vi "Open Handle.vi"(8 "error in (no error)":errorcluster) -> (0 "error out":errorcluster, 3 "Refnum out":T1)   [LabVIEW 2018]
uses:
  <vilib>/httpClient/ClientHandle.ctl
  <vilib>/httpClient/LabVIEWHTTPClient.lvlib
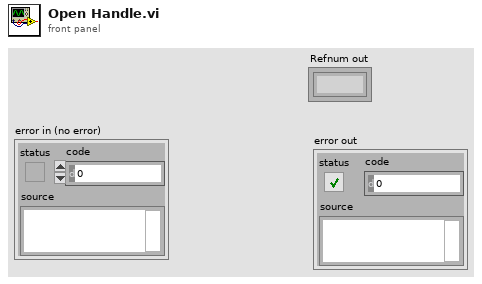
[diagram p1: front panel]
types:
  T1 = typedef "LabVIEWHTTPClient.lvlib/ClientHandle.ctl" = refnum<k1>
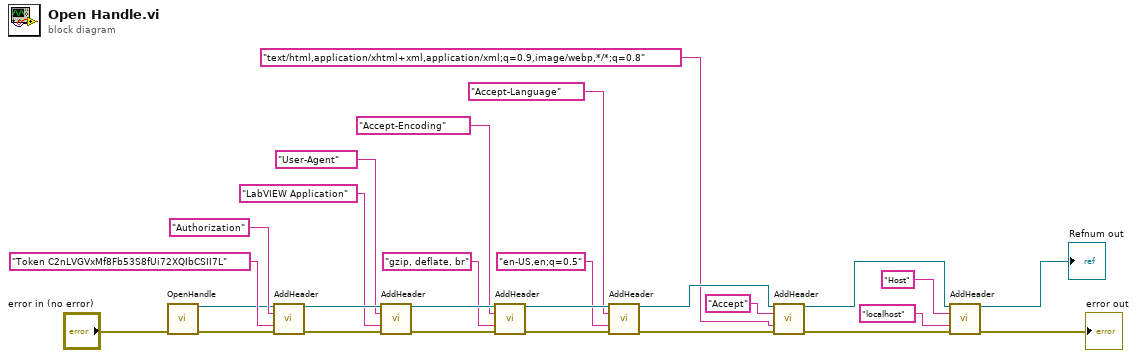
[diagram p0: block diagram]
diagram:
  n1 = call <vilib>:"OpenHandle.vi"("error in (no error)"="error in (no error)") -> ("client handle out"=w2:T1, "error out"=w3:errorcluster)  [unwired: 13 in]
  n2 = call <vilib>:"AddHeader.vi"("client handle"=w2, "header"="Authorization", "value"="Token C2nLVGVxMf8Fb53S8fUi72XQIbCSII7L", "error in (no error)"=w3) -> ("client handle out"=w8:T1, "error out"=w9:errorcluster)  [unwired: 10 in]
  n3 = call <vilib>:"AddHeader.vi"("client handle"=w8, "header"="User-Agent", "value"="LabVIEW Application", "error in (no error)"=w9) -> ("client handle out"=w18:T1, "error out"=w19:errorcluster)  [unwired: 10 in]
  n4 = call <vilib>:"AddHeader.vi"("client handle"=w18, "header"="Accept-Encoding", "value"="gzip, deflate, br", "error in (no error)"=w19) -> ("client handle out"=w16:T1, "error out"=w20:errorcluster)  [unwired: 10 in]
  n5 = call <vilib>:"AddHeader.vi"("client handle"=w16, "header"="Accept-Language", "value"="en-US,en;q=0.5", "error in (no error)"=w20) -> ("client handle out"=w17:T1, "error out"=w21:errorcluster)  [unwired: 10 in]
  n6 = call <vilib>:"AddHeader.vi"("client handle"=w17, "header"="Accept" ("value"), "value"="text/html,application/xhtml+xml,application/xml;q=0.9,image/webp,*/*;q=0.8", "error in (no error)"=w21) -> ("client handle out"=w24:T1, "error out"=w26:errorcluster)  [unwired: 10 in]
  n7 = call <vilib>:"AddHeader.vi"("client handle"=w24, "header"="Host" ("value"), "value"="localhost", "error in (no error)"=w26) -> ("client handle out"=→"Refnum out":T1, "error out"=→"error out":errorcluster)  [unwired: 10 in]
